vi "oa_Process Counter Data (N Tach).vi"(7 "reset?(True)":bool=TRUE, 8 "error in (no error)":errorcluster, 9 "vibration data durations [s]":dbl[](array[numeric]), 11 "digital tach info":T2[](array[typedef])) -> (0 "error out (no error)":errorcluster, 3 "digital tach info out (DBL)":T1(array[cluster]) {"counter timebase [Hz]" format="%.2f"; "pulse positions [s]" format="%.2f"})   [LabVIEW 2017, in "SoundVib_TachProcess.lvlib"]
uses:
  <vilib>/addons/Sound and Vibration/Order Analysis/Tach Process/SoundVib_TachProcess.lvlib
  <vilib>/addons/Sound and Vibration/Order Analysis/Tach Process/SubVIs/digital tach info.ctl
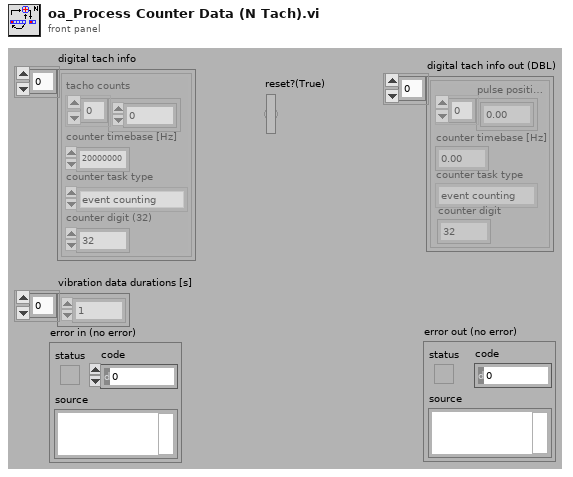
[diagram p1: front panel]
types:
  T1 = cluster{"pulse positions [s]":dbl[], "counter timebase [Hz]":dbl, "counter task type":enum16{"period measurement", "event counting"}, "counter digit":i32}[]
  T2 = typedef "SoundVib_TachProcess.lvlib/digital tach info.ctl" = cluster{"tacho counts":i64[], "counter timebase [Hz]":dbl, "counter task type":enum16{"period measurement", "event counting"}, "counter digit (32)":i32}
  T3 = cluster{"pulse positions [s]":dbl[], "counter timebase [Hz]":dbl, "counter task type":enum16{"period measurement", "event counting"}, "counter digit":i32}
  T4 = cluster{"time offset":dbl, "event count":u64, "time without pulse":ext}
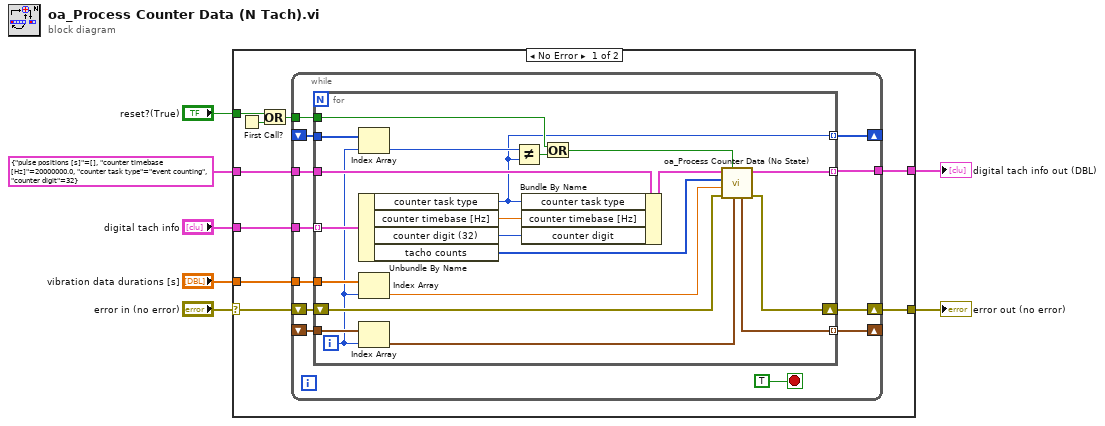
[diagram p0: block diagram]
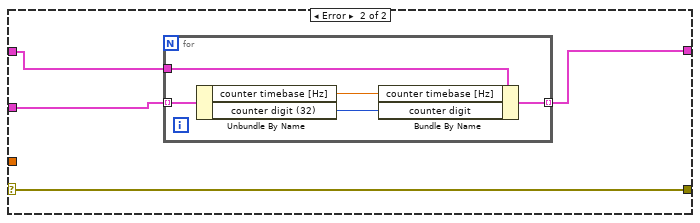
[diagram p2: hidden frame]
diagram:
  n1 = case shown="No Error" "error in (no error)" {
    selector: "error in (no error)" -> [w9 w53]
    tunnel: [w8 w53] -> w6
    tunnel: "digital tach info" -> [w16 w52]
    tunnel: [w12 w51] -> w4
    tunnel: "reset?(True)" -> [w14 _]
    tunnel: "vibration data durations [s]" -> [w11 _]
    tunnel: T3 {"pulse positions [s]"=[], "counter timebase [Hz]"=20000000.0, "counter task type"=enum."event counting", "counter digit"=32} ("digital tach info (DBL)") -> [w10 w50]
    frame No Error {
      n2 = First Call?() -> (First Call?: T/F=w13:bool)
      n3 = Or(x=w14, y=w13) -> (x .or. y?=w15:bool)
      n4 = while {
        tunnel: w15 -> [w28]
        tunnel: [w27] -> w12
        tunnel: w16 -> [w26]
        shift-right: [w25] -> _
        shift-left: _ -> [w24]
        shift-right: [w17] -> _
        shift-left: _ -> [w22]
        tunnel: w11 -> [w21]
        tunnel: w10 -> [w20]
        shift-right: [w18] -> w8
        shift-left: w9 -> [w19]
        stop <- TRUE stop-if-true
        n5 = for {
          tunnel: w26 -> [w47] mode=indexing
          tunnel: w28 -> [w46]
          tunnel: [w38] -> w27 mode=indexing
          tunnel: [w37] -> w25 mode=indexing
          tunnel: w24 -> [w49]
          tunnel: w22 -> [w48]
          tunnel: w21 -> [w33]
          tunnel: w20 -> [w41]
          shift-right: [w34] -> w18
          shift-left: w19 -> [w35]
          tunnel: [w30] -> w17 mode=indexing
          i -> [w32]
          n6 = Index Array(array=w49, index=w32) -> (element=w45:enum16{"period measurement", "event counting"})
          n7 = Unbundle By Name(w47) -> ("counter task type"=w37:enum16{"period measurement", "event counting"}, "counter timebase [Hz]"=w43:dbl, "counter digit (32)"=w44:i32, "tacho counts"=w36:i64[])
          n8 = Index Array(array=w33, index=w32) -> (element=w31:dbl)
          n9 = Index Array(array=w48, index=w32) -> (element=w29:T4)
          n10 = Not Equal?(x=w45, y=w37) -> (x != y?=w42:bool)
          n11 = Bundle By Name(cluster=w41, "counter task type"=w37, "counter timebase [Hz]"=w43, "counter digit"=w44) -> (w39:T3)
          n12 = Or(x=w46, y=w42) -> (x .or. y?=w40:bool)
          n13 = call <vilib>:"oa_Process Counter Data (No State).vi"("state in"=w29, "reset"=w40, "error in (no error)"=w35, "vibration signal duration [s]"=w31, "tacho counts"=w36, "digital tach info in"=w39) -> ("error out"=w34:errorcluster, "digital tach info out"=w38:T3, "state out"=w30:T4)  [unwired: 3 in]
        }
      }
    }
    frame Error {
      n14 = for {
        tunnel: w52 -> [w57] mode=indexing
        tunnel: w50 -> [w58]
        tunnel: [w54] -> w51 mode=indexing
        n15 = Unbundle By Name(w57) -> ("counter timebase [Hz]"=w56:dbl, "counter digit (32)"=w55:i32)
        n16 = Bundle By Name(cluster=w58, "counter timebase [Hz]"=w56, "counter digit"=w55) -> (w54:T3)
      }
    }
  }
  "error out (no error)" <- w6
  "digital tach info out (DBL)" <- w4
